vi "New Ripple A.vi"(11 "GIC Input":T1={"     Use ?\nOff       On"=[FALSE, TRUE, FALSE, TRUE], "Mode:"=FALSE, "Extra Port"="", "Hokuyo Port"="COM7", "Tx Prop  Port"="COM6", "Compass Port"="", "GPS Port"="", "Num of WPs"=0, "WP Lats and Longs"={"WP Lats"=[], "WP Longs"=[]}, "Obst Lats and Longs"={"Obst Lats"=[], "Obst Longs"=[]}, "Parameters"=[], "GPS Data"=[], "Compass"=0.0, "LMS Vector"=[], "Vision Vector"=[], "Direction Cmd"=0.0, "Speed Cmd"=0.0, "WP Vector"=[], "WP Number"=0, "Extra"=0, "SW Map"=[], "Path Cluster"={"Path x node"=[], "Path y node"=[]}, "Sim Course"=[]} {"Obst Lats and Longs"."Obst Longs" format="%#_8g"; "Obst Lats and Longs"."Obst Lats" format="%#_8g"}) -> (3 "GIC Output":T1={"     Use ?\nOff       On"=[FALSE, TRUE, FALSE, TRUE], "Mode:"=FALSE, "Extra Port"="", "Hokuyo Port"="COM7", "Tx Prop  Port"="COM6", "Compass Port"="", "GPS Port"="", "Num of WPs"=0, "WP Lats and Longs"={"WP Lats"=[], "WP Longs"=[]}, "Obst Lats and Longs"={"Obst Lats"=[], "Obst Longs"=[]}, "Parameters"=[], "GPS Data"=[], "Compass"=0.0, "LMS Vector"=[], "Vision Vector"=[], "Direction Cmd"=0.0, "Speed Cmd"=0.0, "WP Vector"=[], "WP Number"=0, "Extra"=0, "SW Map"=[], "Path Cluster"={"Path x node"=[], "Path y node"=[]}, "Sim Course"=[]} {"Obst Lats and Longs"."Obst Longs" format="%#_8g"; "Obst Lats and Longs"."Obst Lats" format="%#_8g"})   [LabVIEW 2014]
panel:
  in  "Test Parameters":dbl[](array[numeric])
  out "Array":dbl[](array[numeric])
  out "test":dbl
  out "Test SWMap Out":dbl[][](array[numeric])
  # "New Ripple A"
  # "Input:"
  # "Output"
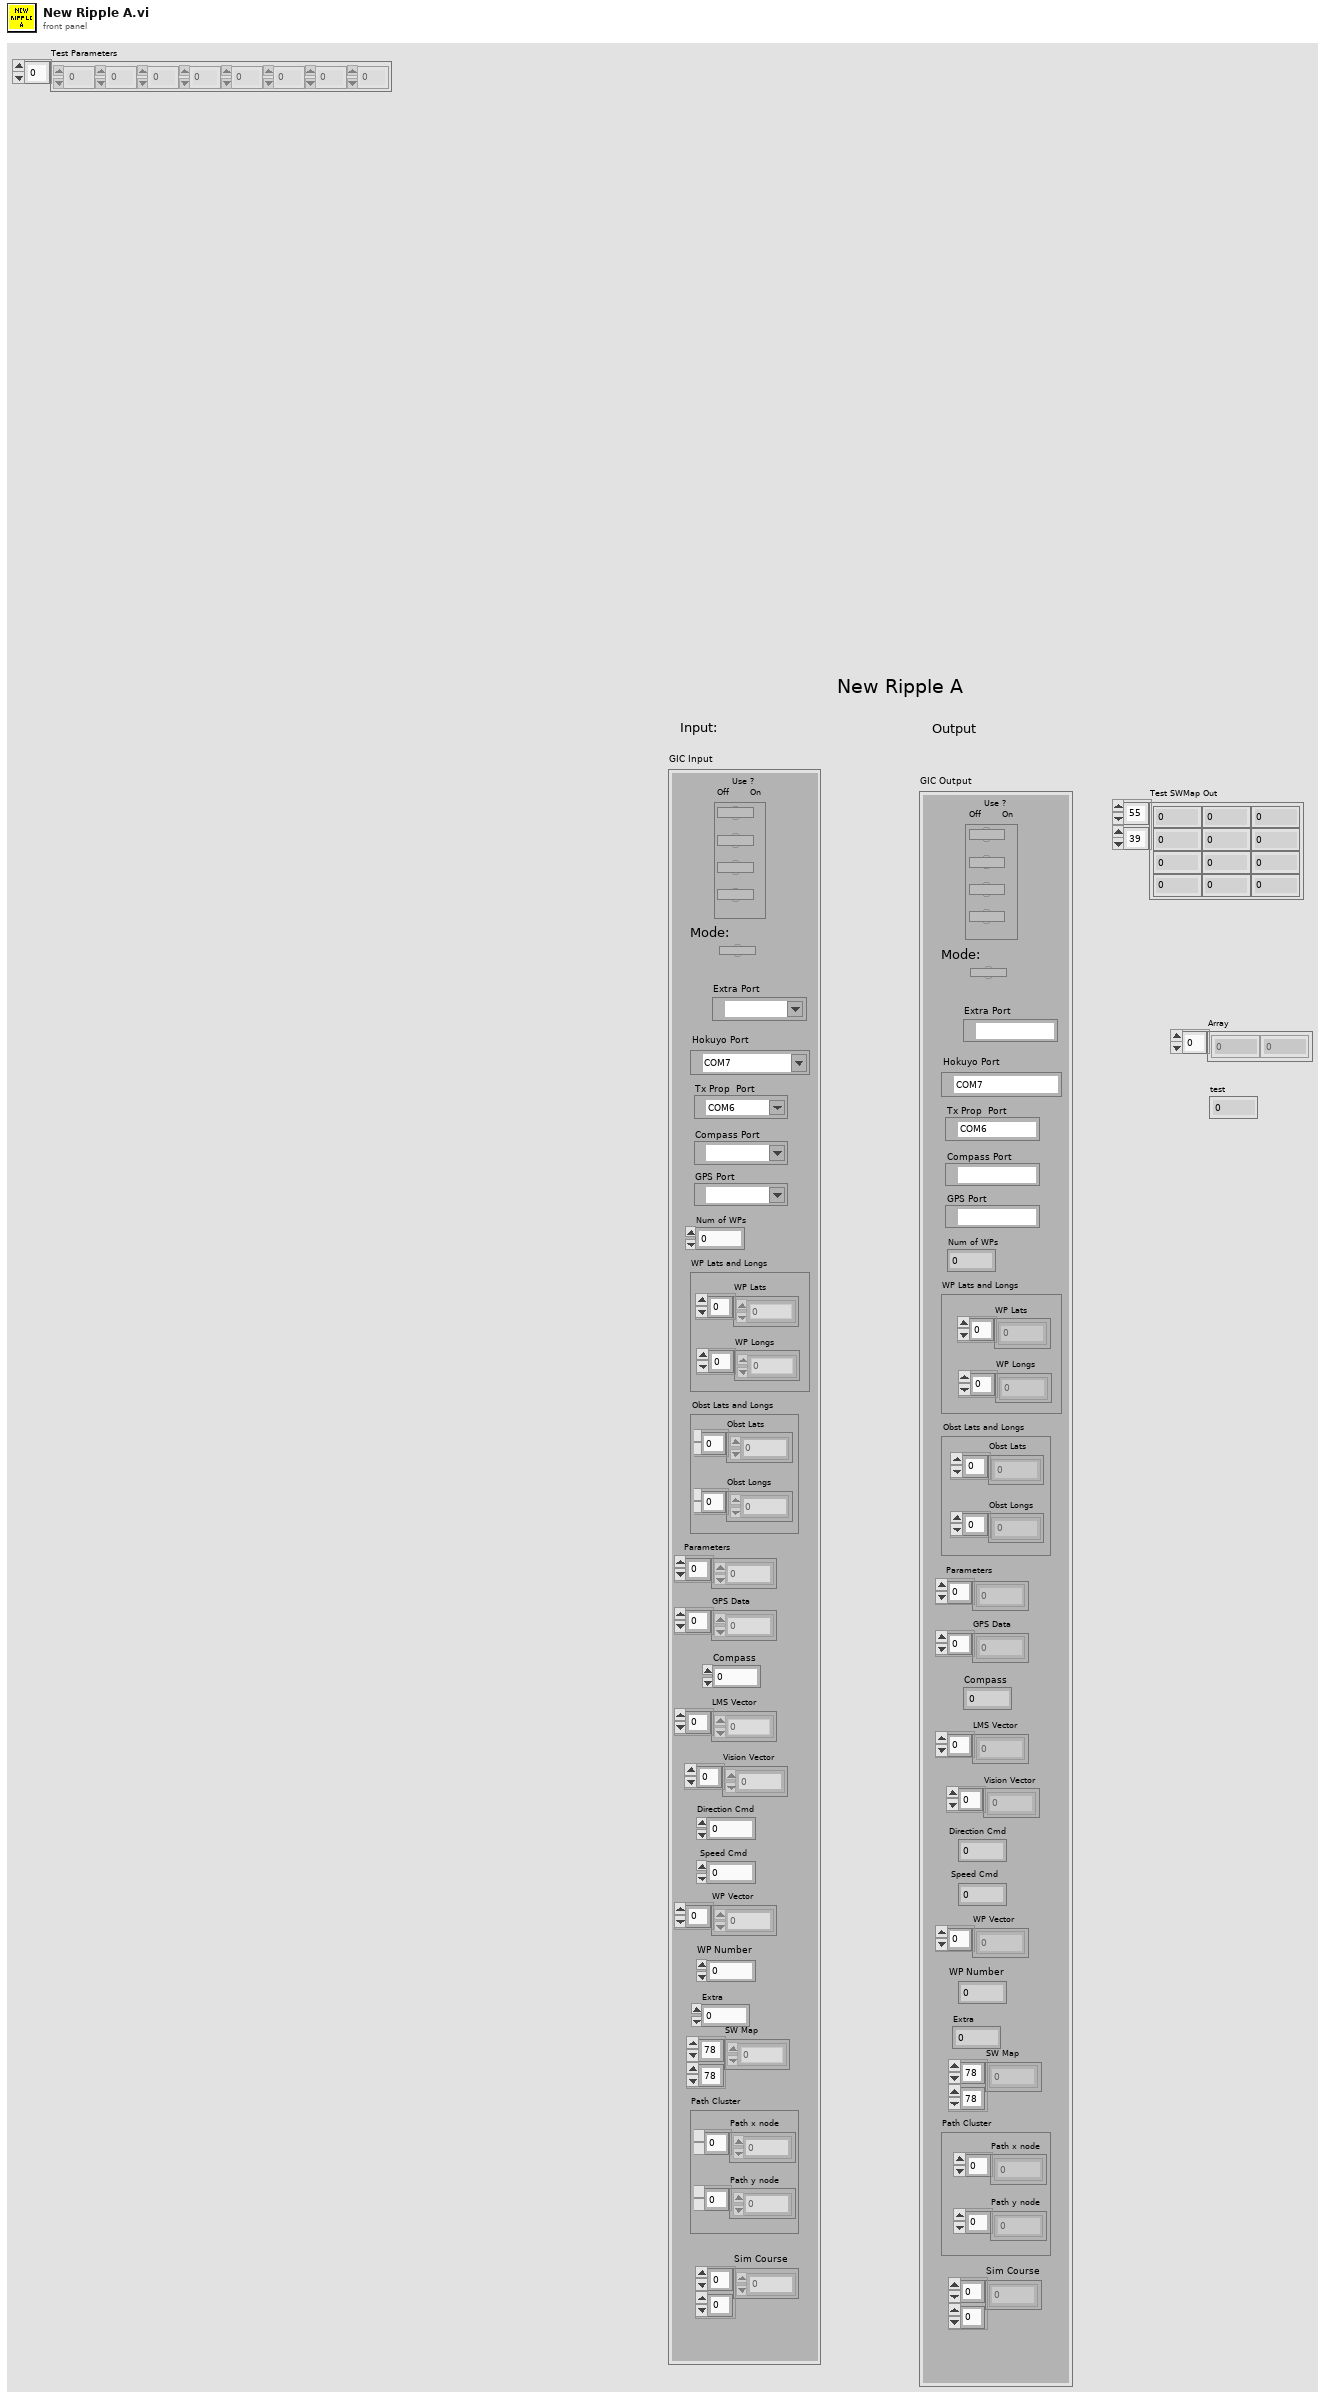
[diagram p1: front panel]
types:
  T1 = cluster{"     Use ?\nOff       On":bool[], "Mode:":bool, "Extra Port":refnum<visa-resource-name>, "Hokuyo Port":refnum<visa-resource-name>, "Tx Prop  Port":refnum<visa-resource-name>, "Compass Port":refnum<visa-resource-name>, "GPS Port":refnum<visa-resource-name>, "Num of WPs":i16, "WP Lats and Longs":cluster{"WP Lats":dbl[], "WP Longs":dbl[]}, "Obst Lats and Longs":cluster{"Obst Lats":dbl[], "Obst Longs":dbl[]}, "Parameters":dbl[], "GPS Data":dbl[], "Compass":dbl, "LMS Vector":dbl[], "Vision Vector":dbl[], "Direction Cmd":dbl, "Speed Cmd":dbl, "WP Vector":dbl[], "WP Number":i32, "Extra":i16, "SW Map":i32[][], "Path Cluster":cluster{"Path x node":dbl[], "Path y node":dbl[]}, "Sim Course":i8[][]}
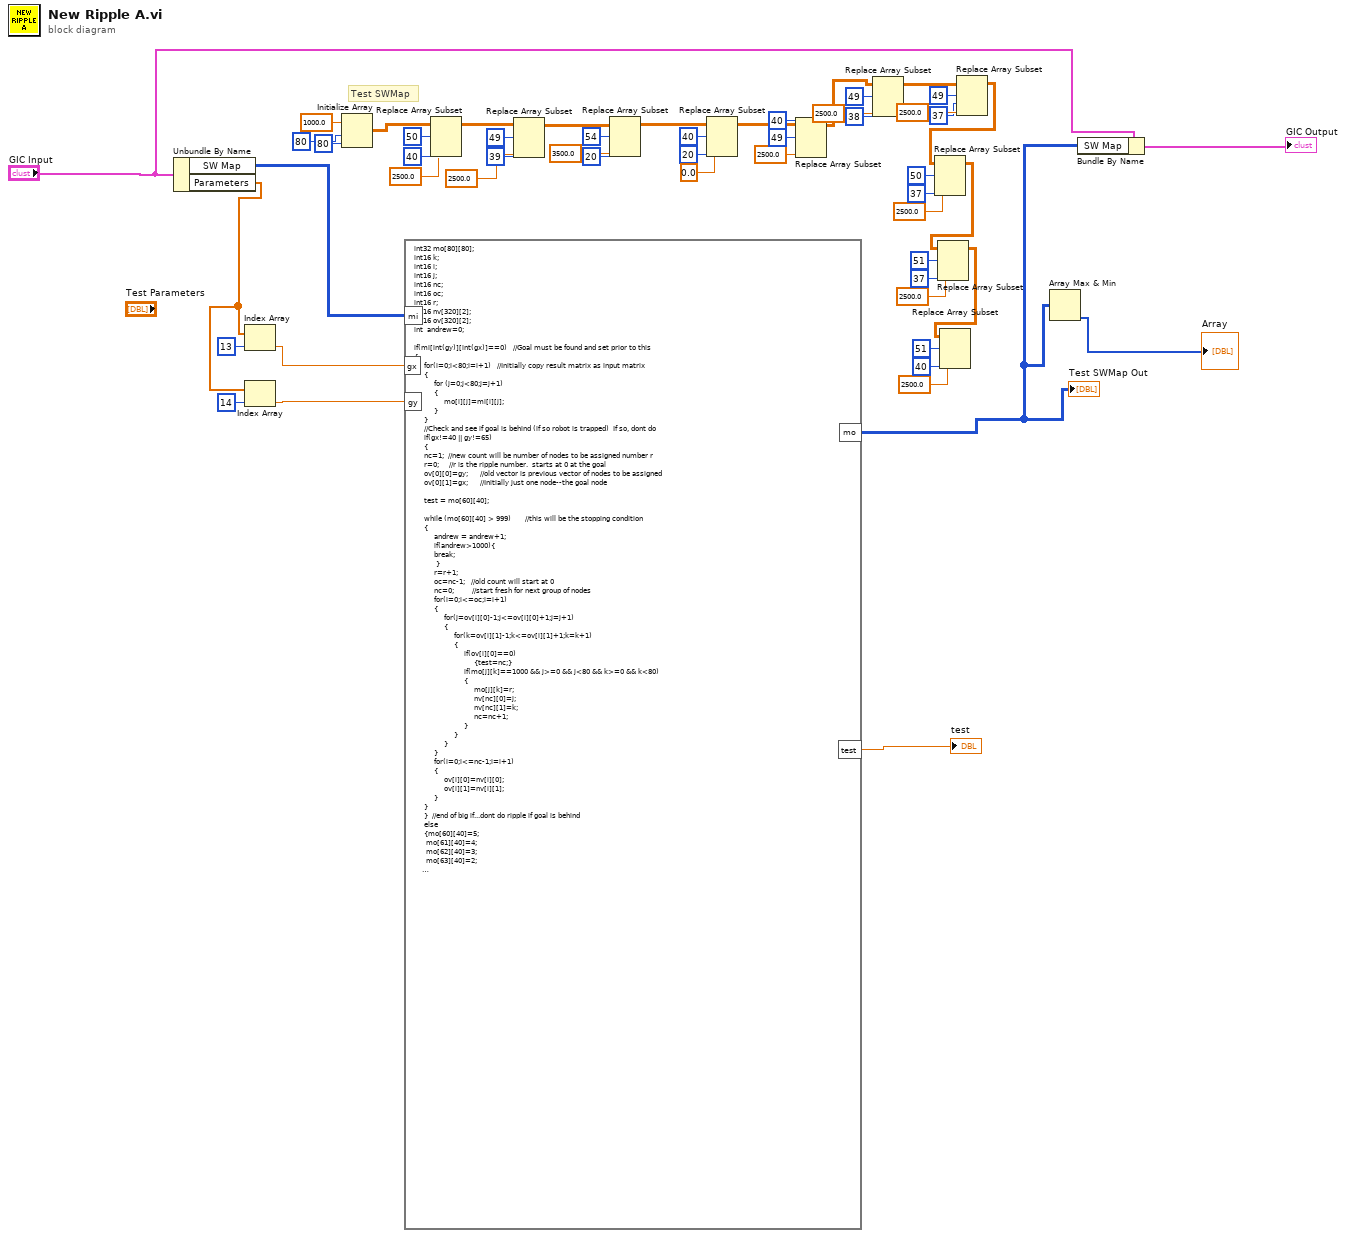
[diagram p0: block diagram]
diagram:
  # "Test SWMap"
  n1 = Unbundle By Name("GIC Input") -> ("SW Map"=w3:i32[][], "Parameters"=w4:dbl[])
  n2 = Index Array(array=w4, index=13) -> (element=w33:dbl)
  n3 = Index Array(array=w4, index=14) -> (element=w30:dbl)
  n4 = Initialize Array(1000.0 ("element"), 80 ("dimension size"), 80 ("dimension size")) -> (w51:dbl[][])
  n5 = formula code="int32 mo[80][80];\nint16 k;\nint16 i;\nint16 j;\nint16 nc;\nint16 oc;\nint16 r;\nint16 nv[320][2];\nint16 ov[320][2];\nint  andrew=0;\n\nif(mi[int(gy)][int(gx)]==0)   //Goal must be found and set prior to this\n{\n     for(i=0;i<80;i=i+1)   //Initially copy result matrix as input matrix\n     {\n          for (j=0;j<80;j=j+1)\n          {\n               mo[i][j]=mi[i][j];\n          }\n     }\n     //Check and see if goal is behind (if so robot is trapped)  If so, dont do\n     if(gx!=40 || gy!=65)\n     {\n     nc=1;  //new count will be number of nodes to be assigned number r\n     r=0;     //r is the ripple number.  starts at 0 at the goal\n     ov[0][0]=gy;      //old vector is previous vector of nodes to be assigned\n     ov[0][1]=gx;      //Initially just one node--the goal node\n\n     test = mo[60][40];\n\n     while (mo[60][40] > 999)       //this will be the stopping condition\n     {\n          andrew = andrew+1;\n          if(andrew>1000){\n          break;\n           }\n          r=r+1;\n          oc=nc-1;   //old count will start at 0\n          nc=0;         //start fresh for next group of nodes\n          for(i=0;i<=oc;i=i+1)\n          {\n               for(j=ov[i][0]-1;j<=ov[i][0]+1;j=j+1)\n               {\n                    for(k=ov[i][1]-1;k<=ov[i][1]+1;k=k+1)\n                    {\n                         if(ov[i][0]==0)\n                              {test=nc;}\n                         if(mo[j][k]==1000 && j>=0 && j<80 && k>=0 && k<80)\n                         {\n                              mo[j][k]=r;\n                              nv[nc][0]=j;\n                              nv[nc][1]=k;\n                              nc=nc+1;\n                         }\n                    }\n               }\n          }\n          for(i=0;i<=nc-1;i=i+1)\n          {\n               ov[i][0]=nv[i][0];\n               ov[i][1]=nv[i][1];\n          }\n     }\n     }  //end of big if...dont do ripple if goal is behind\n     else\n     {mo[60][40]=5;\n      mo[61][40]=4;\n      mo[62][40]=3;\n      mo[63][40]=2;\n      mo[64][40]=1;}\n}"("mi"=w3, "gx"=w33, "gy"=w30) -> ("mo"=w38:i32[][], "test"=→"test":dbl)
  "Test SWMap Out" <- w38
  n6 = Replace Array Subset(array=w51, new element=2500.0 ("new element/subarray"), index (row)=50, index (col)=40 ("disabled index (col)")) -> (w47:dbl[][])
  n7 = Replace Array Subset(array=w47, new element=2500.0 ("new element/subarray"), index (row)=49, index (col)=39 ("disabled index (col)")) -> (w42:dbl[][])
  n8 = Replace Array Subset(array=w42, new element=3500.0 ("new element/subarray"), index (row)=54, index (col)=20 ("disabled index (col)")) -> (w37:dbl[][])
  n9 = Replace Array Subset(array=w37, new element=0.0 ("new element/subarray"), index (row)=40, index (col)=20 ("disabled index (col)")) -> (w28:dbl[][])
  n10 = Replace Array Subset(array=w28, new element=2500.0 ("new element/subarray"), index (row)=49, index (col)=40 ("disabled index (col)")) -> (w24:dbl[][])
  n11 = Replace Array Subset(array=w24, new element=2500.0 ("new element/subarray"), index (row)=49, index (col)=38 ("disabled index (col)")) -> (w20:dbl[][])
  n12 = Replace Array Subset(array=w20, new element=2500.0 ("new element/subarray"), index (row)=49, index (col)=37 ("disabled index (col)")) -> (w16:dbl[][])
  n13 = Replace Array Subset(array=w16, new element=2500.0 ("new element/subarray"), index (row)=50, index (col)=37 ("disabled index (col)")) -> (w12:dbl[][])
  n14 = Replace Array Subset(array=w12, new element=2500.0 ("new element/subarray"), index (row)=51, index (col)=37 ("disabled index (col)")) -> (w8:dbl[][])
  n15 = Replace Array Subset(array=w8, new element=2500.0 ("new element/subarray"), index (row)=51, index (col)=40 ("disabled index (col)")) -> ()  [unwired: 1 out]
  n16 = Array Max & Min(array=w38) -> (min index (indices)=→"Array":i32[])  [unwired: 3 out]
  n17 = Bundle By Name(cluster="GIC Input", "SW Map"=w38) -> (→"GIC Output":T1)
